vi "chaosui-crest-cu-get-channel.vi"(8 "handleConnection":T2, 9 "channame":string, 10 "cuname":string, 11 "timeout (10000)":i32=10000) -> (3 "timestamp":u64, 4 "nok":i32, 5 "value out":string)   [LabVIEW 2014]
doc: "uint64_t chaos_crest_cu_get_channel(chaos_crest_handle_t h,const char*cuname,const char*channame,char*output,int maxsize);"
uses:
  chaosui-crest.lvlib
  <vilib>/httpClient/ClientHandle.ctl
  <vilib>/httpClient/LabVIEWHTTPClient.lvlib
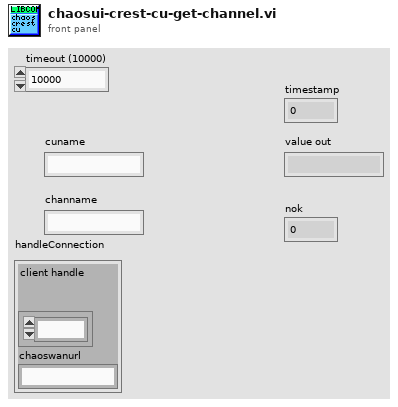
[diagram p1: front panel]
types:
  T1 = typedef "LabVIEWHTTPClient.lvlib/ClientHandle.ctl" = refnum<k1>
  T2 = cluster{"client handle":T1, "chaoswanurl":string}
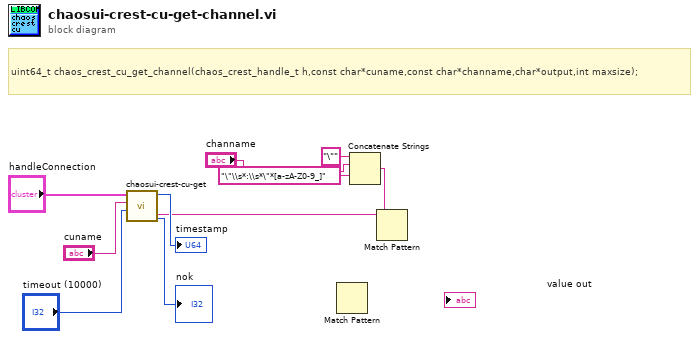
[diagram p0: block diagram]
diagram:
  # "uint64_t chaos_crest_cu_get_channel(chaos_crest_handle_t h,const char*cuname,const char*channame,char*output,int maxsize);"
  n1 = call "chaosui-crest-cu-get.vi"("timeout (10000)"="timeout (10000)", "cuname"="cuname", "handleConnection"="handleConnection") -> ("nok"=→"nok":i32, "timestamp"=→"timestamp":u64, "output out"=w6:string)  [unwired: 1 in, 2 out]
  n2 = Match Pattern() -> ()  [unwired: 3 in, 4 out]
  n3 = Concatenate Strings("\"" ("string"), "channame", "\"\\s*:\\s*\"*[a-zA-Z0-9_]" ("string")) -> (w1:string)  [unwired: 1 in]
  n4 = Match Pattern(string=w6, regular expression=w1) -> ()  [unwired: 1 in, 4 out]
